vi "MGCC_FntStaMach_gobal.vi"() -> ()   [LabVIEW 2016]
doc: "-----------------------------------------------------------------------------------------------------------------------\nCopyright <2019> <The University of Tennessee at Knoxville and the University of Tennessee Research Foundation>\nThis software is released under BSD-3 \nhttps://opensource.org/licenses/BSD-3-Clause \nAdditional license options available at https://utrf.tennessee.edu/industry/sample-agreements/\n-----------------------------------------------------------------------------------------------------------------------"
panel:
  in  "b_MGCC_FntStaMach_IsdCon_enable":bool
  in  "b_MGCC_FntStaMach_Resync_Enable":bool
  in  "b_MGCC_FntStaMach_BlkStart_Enable":bool
  in  "b_MGCC_FntStaMach_UnplannedISD_enable":bool
  in  "b_MGCC_FntStaMach_PlanISD_enable":bool
  in  "b_MGCC_FntStaMach_DataLog_enable":bool
  in  "b_MGCC_FntStaMach_PVFcst_Enable":bool
  in  "b_MGCC_FntStaMach_EnergyMgmt_Enable":bool
  in  "b_MGCC_FntStaMach_LoadFcst_Enable":bool
  in  "b_MGCC_FntStaMach_PQBal_enable":bool
  in  "b_MGCC_FntStaMach_state_estimation_enable":bool
  in  "Enable":bool[](array[boolean])
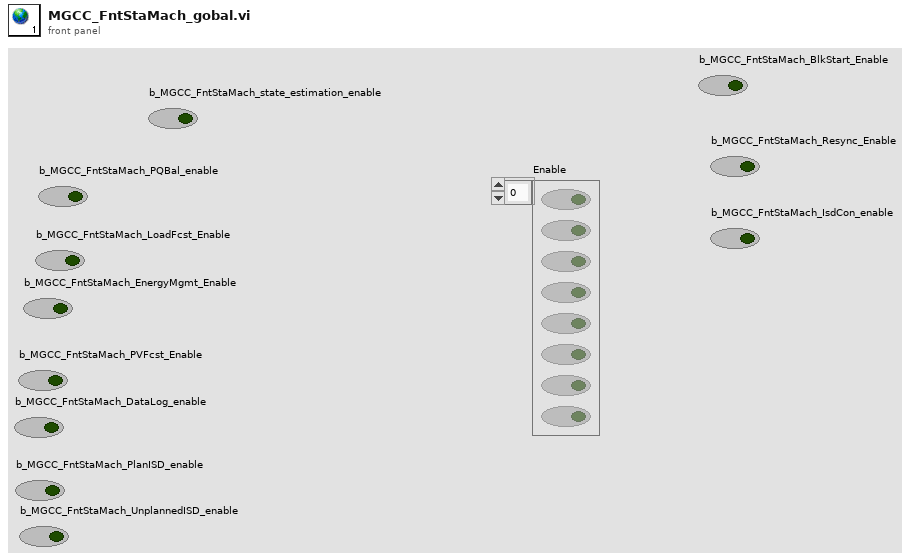
[diagram p1: front panel]
diagram:
